vi "test.vi"(5 "Coupling":u16(ring)=2 items=["DC 1 MOhm", "AC 1 MOhm", "DC 50 Ohm", "AC 50 OHM"], 6 "RF data Sampling":T2={"Sampling Rate"=0, "Delay (micro s)"=0.0, "rf points per line"=500} {"Delay (micro s)" format="%.2f"}, 7 "Boolean":bool) -> (0 "voltage range":T1, 1 "Equivalent delay\ndistance (mm)":dbl=1.5 format="%.2f", 2 "RF data Out":T2 {"Delay (micro s)" format="%.2f"}, 3 "ID":i32)   [LabVIEW 2022 SP3]
uses:
  Instance          14 12Saved   test .vi
  Instance          15 12Saved   test .vi
  <instrlib>/Acqiris Bx/Acqiris Bx.lvlib
  <instrlib>/Acqiris Dx/Acqiris Dx.lvlib
panel:
  out "Nominal Samples":i32
  out "Samping Rate":dbl format="%.2f"
  in  "ExitSendCmd":bool
  out "instrumentID":u32
  in  "Voltage Full Scale (pp)":u16(ring)=3
  in  "Time scale per Div":i32(ring)=8 items=["1 ns", "5 ns", "10 ns", "20 ns", "50 ns", "100 ns", "200 ns", "500 ns", "1 micros", "2 micros", "5 micros", "10 micros", "20 micros", "50 micros", "100 micros", "200 micros", "500 micros", "1 ms", "2 ms", "5 ms", "10 ms", "20 ms", "50 ms", "100 ms", "200 ms"]
  out "Waveform Graph":cluster{i32, dbl, "Acquired Waveform SGL":dbl[]}(graph)
  out "errorMessage":string
  in  "Trigger":T3={"Source"=1, "Coupling"=0, "Slope"=0, "Level (% CH1 or mV Ext)"=1000.0} {"Slope" items=["Positive", "Negative"]; "Level (% CH1 or mV Ext)" format="%.2f"; "Coupling" items=["DC 1 MOhm", "AC 1 MOhm", "DC 50 Ohm", "AC 50 Ohm"]; "Source" items=["Chan 1", "External"]}
  # "Take out option of changing offset.  Move in time scale selector."
  # "Red line indicates last pt of RF data"
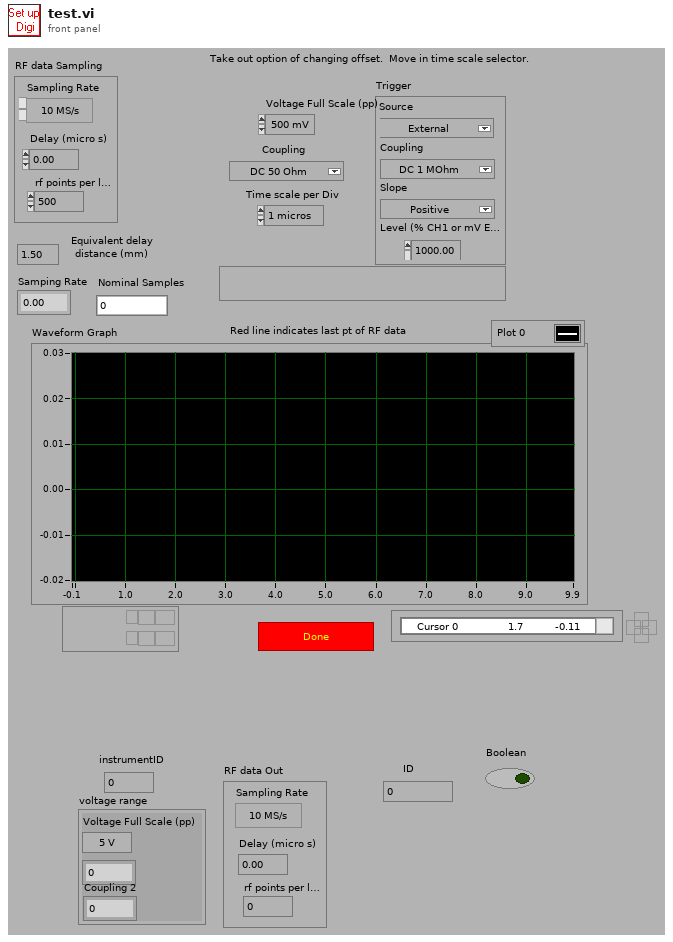
[diagram p1: front panel]
types:
  T1 = cluster{"Voltage Full Scale (pp)":u16, i32, "Coupling 2":u16}
  T2 = cluster{"Sampling Rate":u16, "Delay (micro s)":dbl, "rf points per line":u16}
  T3 = cluster{"Source":u16, "Coupling":u16, "Slope":u16, "Level (% CH1 or mV Ext)":dbl}
  T4 = cluster{"Voltage Full Scale (pp)":u16, i32, "Coupling":u16}
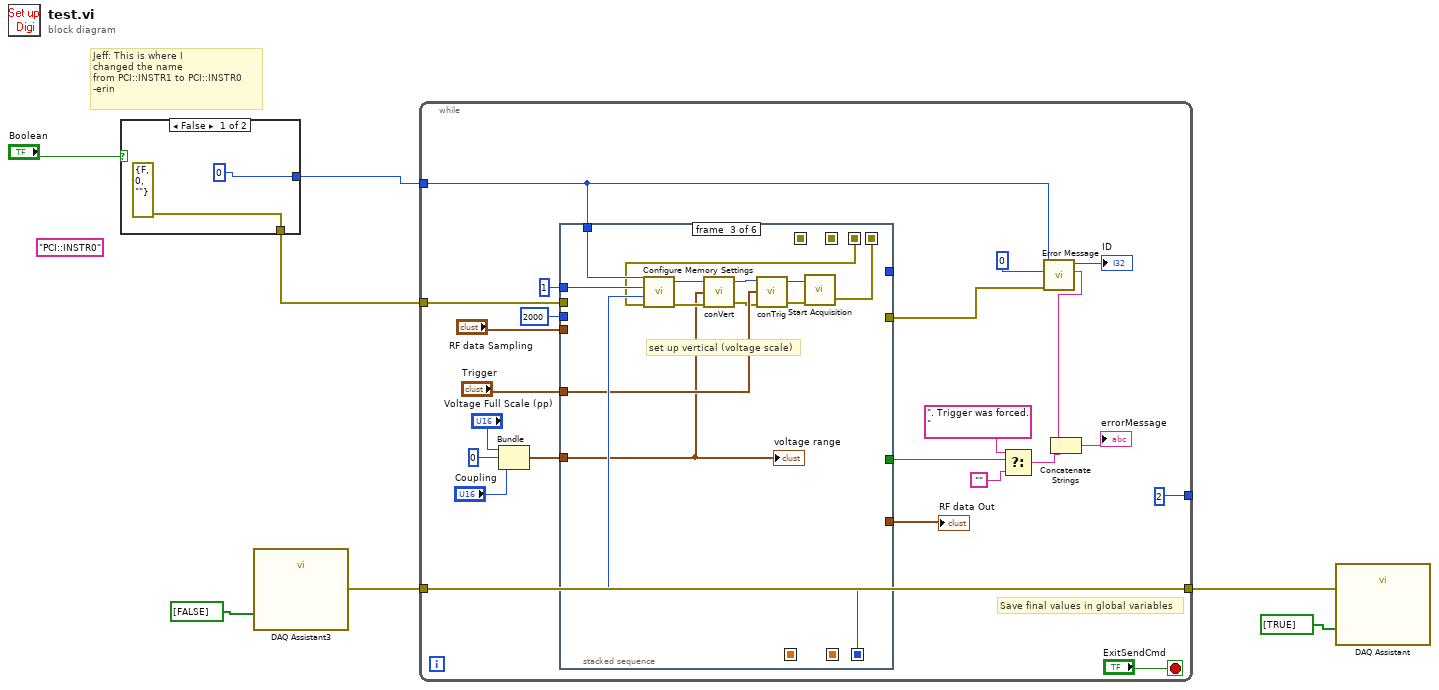
[diagram p0: block diagram]
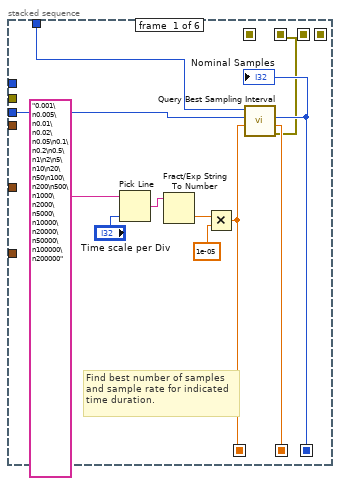
[diagram p2: hidden frame]
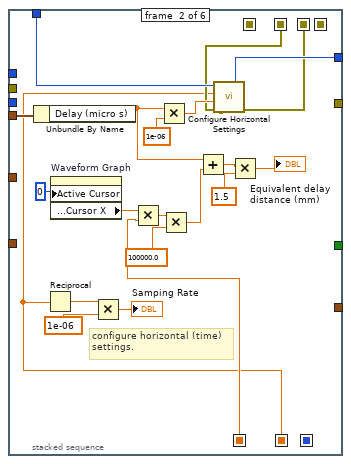
[diagram p3: hidden frame]
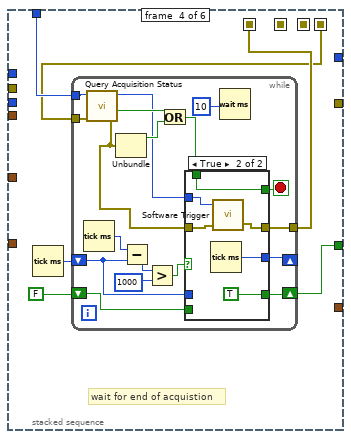
[diagram p4: hidden frame]
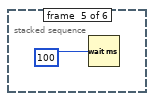
[diagram p6: hidden frame]
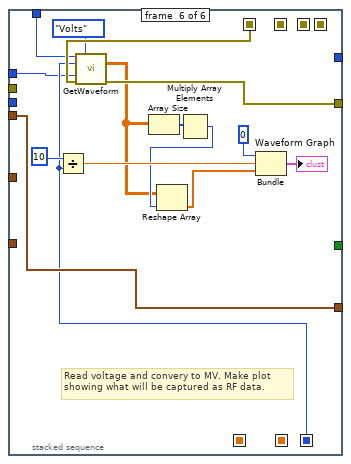
[diagram p7: hidden frame]
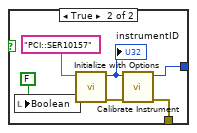
[diagram p8: hidden frame]
diagram:
  (unwired) "PCI::INSTR0" ("resourceName")
  # "Jeff: This is where I \nchanged the name \nfrom PCI::INSTR1 to PCI::INSTR0\n-erin"
  n1 = case shown="False" "Boolean" {
    tunnel: [u32 0 ("dup Instrument ID") w12] -> w6
    tunnel: [errorcluster {"status"=FALSE, "code"=0, "source"=""} ("error out") w14] -> w7
    frame False {
    }
    frame True {
      n2 = local write "Boolean"(FALSE) -> ()
      n3 = call <instrlib>:"Initialize with Options.vi"("Resource Name (PCI::INSTR0)"="PCI::SER10157" ("ResourceName")) -> ("Instrument ID"=w13:u32, "error out"=w15:errorcluster)  [unwired: 5 in, 2 out]
      "instrumentID" <- w13
      n4 = call <instrlib>:"Calibrate Instrument.vi"("error in (no error)"=w15, "Instrument ID"=w13) -> ("error out"=w14:errorcluster, "dup Instrument ID"=w12:u32)  [unwired: 4 out]
    }
  }
  n5 = call "DAQ Assistant3"("data"=bool[] [FALSE]) -> ("error out"=w3:errorcluster)  [unwired: 3 in, 15 out]
  n6 = while {
    tunnel: w7 -> [w30]
    tunnel: w6 -> [w29]
    tunnel: [2] -> _
    tunnel: [w16] -> w2
    tunnel: w3 -> [w16]
    stop <- "ExitSendCmd" stop-if-true
    # "Save final values in global variables"
    n7 = Bundle("Voltage Full Scale (pp)"="Voltage Full Scale (pp)", 0, "Coupling"="Coupling") -> (w19:T4)  [unwired: 1 out]
    n8 = stacked-sequence {
      seq-local: [w42 _ _ _ _ _] -> [_ w53 _ _ _ _]
      seq-local: [w43 _ _ _ _ _] -> [_ _ w80 _ _ w122]
      seq-local: [w40 _ _ _ _ _] -> [_ w65 _ _ _ _]
      seq-local: [_ w64 _ _ _ _] -> [_ _ w79 _ _ _]
      seq-local: [_ _ w74 _ _ _] -> [_ _ _ w84 _ _]
      seq-local: [_ _ _ w85 _ _] -> [_ _ _ _ _ w125]
      seq-local: [w39 _ _ _ _ _] -> [_ w54 _ _ _ _]
      tunnel: w29 -> [w44 w70 w83 w88 _ w123]
      tunnel: [_ w69 _ _ _ _] -> _
      tunnel: "RF data Sampling" -> [_ w67 _ _ _ w129]
      tunnel: [_ _ _ _ _ w129] -> w38
      tunnel: [_ _ _ w86 _ _] -> w32
      tunnel: "Trigger" -> [_ _ w77 _ _ _]
      tunnel: 1 -> [_ _ w81 _ _ w120]
      tunnel: 2000 -> [w41 _ _ _ _ _]
      tunnel: w30 -> [_ _ _ _ _ _]
      tunnel: w19 -> [_ _ w71 _ _ _]
      tunnel: [_ _ _ _ _ w124] -> w28
      frame #0 {
        # "Find best number of samples\nand sample rate for indicated\ntime duration."
        n9 = Pick Line(multi-line string="0.001\n0.005\n0.01\n0.02\n0.05\n0.1\n0.2\n0.5\n1\n2\n5\n10\n20\n50\n100\n200\n500\n1000\n2000\n5000\n10000\n20000\n50000\n100000\n200000" ("ResourceName"), line index="Time scale per Div") -> (output string=w49:string)  [unwired: 1 out]
        n10 = Fract/Exp String To Number(string=w49) -> (number=w47:dbl)  [unwired: 1 in, 3 out]
        n11 = Multiply(x=w47, y=1e-05) -> (x*y=w39:dbl)
        n12 = call <instrlib>:"Query Best Sampling Interval.vi"("Time Window (1E-6 s)"=w39, "Maximum Samples (10000)"=w41, "Instrument ID"=w44) -> ("error out"=w40:errorcluster, "Sampling Interval (s)"=w42:dbl, "Nominal Samples"=w43:i32)  [unwired: 1 in, 1 out]
        "Nominal Samples" <- w43
      }
      frame #1 {
        # "configure horizontal (time)\nsettings."
        n13 = Unbundle By Name(w67) -> ("Delay (micro s)"=w59:dbl)
        n14 = Reciprocal(x=w53) -> (1/x=w52:dbl)
        n15 = property on="Waveform Graph" class="WFGraph (strict)"("Active Cursor"=0) -> ("Cursor.Cursor Position:Cursor X"=w56:dbl)  [unwired: 2 in, 2 out]
        n16 = Multiply(x=w52, y=1e-06) -> (x*y=→"Samping Rate":dbl)
        n17 = Multiply(x=w56, y=w54) -> (x*y=w62:dbl)
        n18 = Multiply(x=w59, y=1e-06) -> (x*y=w66:dbl)
        n19 = Multiply(x=w62, y=100000.0) -> (x*y=w55:dbl)
        n20 = Add(x=w59, y=w55) -> (x+y=w58:dbl)
        n21 = call <instrlib>:"Configure Horizontal Settings.vi"("error in (no error)"=w65, "Delay Time (0 s)"=w66, "Sampling Interval (10 ns)"=w53, "Instrument ID"=w70) -> ("error out"=w64:errorcluster, "dup Instrument ID"=w69:u32)  [unwired: 2 out]
        n22 = Multiply(x=w58, y=1.5) -> (x*y=→"Equivalent delay\ndistance (mm)":dbl)
      }
      frame #2 {
        # "set up vertical (voltage scale)"
        n23 = call <instrlib>:"Configure Memory Settings.vi"("error in (no error)"=w79, "Number of Samples (1000)"=w80, "Number of Segments (1)"=w81, "Instrument ID"=w83) -> ("error out"=w78:errorcluster, "dup Instrument ID"=w82:u32)  [unwired: 2 out]
        n24 = call "conVert.vi"("InstrumentID"=w82, "V scale"=w71, "error in"=w78) -> ("Status"=w73:i32, "error out"=w72:errorcluster)  [unwired: 1 in, 2 out]
        n25 = call "conTrig.vi"("error in"=w72, "Trigger"=w77, "InstrumentID"=w73) -> ("error out"=w76:errorcluster, "dup id"=w75:u32)  [unwired: 2 in]
        n26 = call <instrlib>:"Start Acquisition.vi"("error in (no error)"=w76, "Instrument ID"=w75) -> ("error out"=w74:errorcluster)  [unwired: 2 in, 1 out]
        "voltage range" <- w71
      }
      frame #3 {
        # "wait for end of acquistion"
        n27 = Tick Count (ms)() -> (millisecond timer value=w89:u32)
        n28 = while {
          shift-left: FALSE -> [w99]
          shift-right: [w100] -> w86
          shift-left: w89 -> [w102]
          shift-right: [w103] -> _
          tunnel: w88 -> [w91]
          tunnel: [w97] -> w85
          tunnel: w84 -> [w92]
          stop <- w101 stop-if-true
          n29 = Tick Count (ms)() -> (millisecond timer value=w107:u32)
          n30 = call <instrlib>:"Query Acquisition Status.vi"("error in (no error)"=w92, "Instrument ID"=w91) -> ("error out"=w98:errorcluster, "Done?"=w96:bool, "dup Instrument ID"=w90:u32)  [unwired: 3 out]
          n31 = Unbundle(w98) -> ("status"=w94:bool)  [unwired: 2 out]
          n32 = Subtract(x=w107, y=w102) -> (x-y=w105:u32)
          n33 = Greater?(x=w105, y=1000) -> (0:w106:bool)
          n34 = Or(x=w96, y=w94) -> (x .or. y?=w95:bool)
          n35 = case shown="True" w106 {
            tunnel: w90 -> [_ w117]
            tunnel: [w111 w116] -> w103
            tunnel: w102 -> [w111 _]
            tunnel: [w110 w112] -> w101
            tunnel: w95 -> [w110 w112]
            tunnel: [w109 TRUE] -> w100
            tunnel: w99 -> [w109 _]
            tunnel: w98 -> [w108 w114]
            tunnel: [w108 w113] -> w97
            frame False {
            }
            frame True {
              n36 = Tick Count (ms)() -> (millisecond timer value=w116:u32)
              n37 = call <instrlib>:"Software Trigger.vi"("error in (no error)"=w114, "Instrument ID"=w117) -> ("error out"=w113:errorcluster)  [unwired: 2 out]
            }
          }
          n38 = Wait (ms)(milliseconds to wait=10) -> ()  [unwired: 1 out]
        }
      }
      frame #4 {
        n39 = Wait (ms)(milliseconds to wait=100) -> ()  [unwired: 1 out]
      }
      frame #5 {
        # "Read voltage and convery to MV. Make plot\nshowing what will be captured as RF data."
        n40 = Divide(x=10, y=w122) -> (x/y=w130:dbl)
        n41 = call "GetWaveform.vi"("Acq ID Out"=w123, "Read Mode"=enum32{"ADC", "Volts"}."Volts", "Num Samps"=w122, "Num Segs"=w120, "error in"=w125) -> ("Acquired Waveform SGL"=w121:dbl[][], "error out"=w124:errorcluster)  [unwired: 1 in, 8 out]
        n42 = Array Size(array=w121) -> (size(s)=w128:i32[])
        n43 = Multiply Array Elements(1:w128) -> (0:w127:i32)
        n44 = Reshape Array(w121, w127) -> (w126:dbl[])
        n45 = Bundle(0, w130, "Acquired Waveform SGL"=w126) -> (→"Waveform Graph":cluster{i32, dbl, "Acquired Waveform SGL":dbl[]})  [unwired: 1 out]
      }
    }
    "RF data Out" <- w38
    n46 = Select(t=". Trigger was forced.", s=w32, f="") -> (s? t:f=w34:string)
    n47 = call <instrlib>:"Error Message.vi"("Instrument ID"=w29, "Type of Dialog (1: OK Msg)"=0, "error in (no error)"=w28) -> ("dup Instrument ID"=→"ID":u32, "Error Message"=w37:string)  [unwired: 5 out]
    n48 = Concatenate Strings(w37, w34) -> (→"errorMessage":string)
  }
  n49 = call "DAQ Assistant"("data"=bool[] [TRUE], "error in"=w2) -> ()  [unwired: 2 in, 16 out]
